vi "移位寄存器.vi"() -> ()   [LabVIEW 2020]
doc: "本VI是为《我和LabVIEW》一书编写的示例。\n关于本书的介绍请参考网页：\nhttp://ruanqizhen.spaces.live.com/blog/cns!5852D4F797C53FB6!4310.entry"
panel:
  out "最后一次迭代的结果":i32
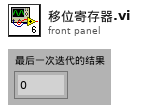
[diagram p1: front panel]
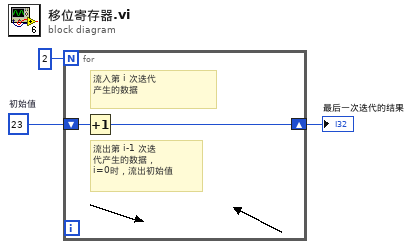
[diagram p0: block diagram]
diagram:
  w3 = 23  # 初始值
  n1 = for {
    N: 2 -> [_]
    shift-right: [w4] -> w2
    shift-left: w3 -> [w5]
    # "流出第 i-1 次迭\n代产生的数据，\ni=0时，流出初始值"
    # "流入第 i 次迭代\n产生的数据"
    n2 = Increment(x=w5) -> (x+1=w4:i32)
  }
  "最后一次迭代的结果" <- w2
